vi "test.vi"() -> ()   [LabVIEW 2023]
uses:
  <vilib>/Instr/_visa.llb/VISA Configure Serial Port (Instr).vi
panel:
  out "read buffer 2":string
  out "read buffer":string
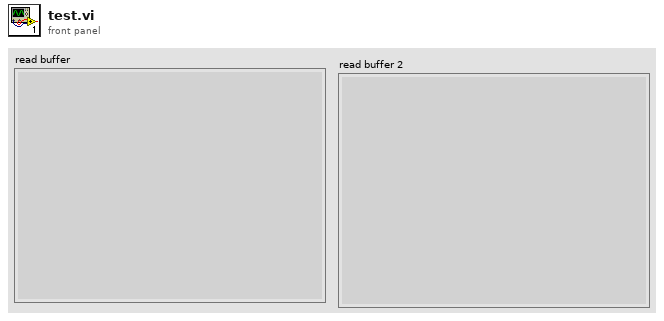
[diagram p1: front panel]
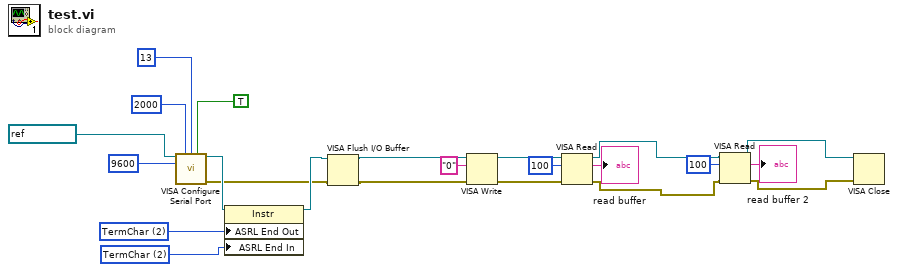
[diagram p0: block diagram]
diagram:
  w18 = u16 2 items=["None", "Last Bit", "TermChar", "Break"] ("Serial Settings:End Mode for Writes")
  w17 = u16 2 items=["None", "Last Bit", "TermChar", "Break"] ("Serial Settings:End Mode for Writes")
  n1 = call-poly "VISA Configure Serial Port"("VISA resource name"=refnum<visa-resource-name> "COM10", "timeout (10sec)"=u32 2000, "termination char\n(0xA = '\\n' = LF)"=u8 13 ("termination char\n(0xA = '\\n' = LF)"), "Enable Termination\nChar (T)"=TRUE ("Enable Termination\nChar (T)"), "baud rate (9600)"=u32 9600) -> ("VISA resource name out"=w19:refnum<visa-resource-name>, "error out"=w2:errorcluster)  [unwired: 9 in]
  n2 = property class="Instr"(reference=w19, "ASRL End Out"=w18, "ASRL End In"=w17) -> (reference out=w5:refnum<visa-resource-name>)  [unwired: 1 in, 1 out]
  n3 = VISA Flush I/O Buffer(VISA resource name=w5, error in (no error)=w2) -> (VISA resource name out=w4:refnum<visa-resource-name>, error out=w3:errorcluster)  [unwired: 1 in]
  n4 = VISA Write(VISA resource name=w4, write buffer="0", error in (no error)=w3) -> (VISA resource name out=w15:refnum<visa-resource-name>, error out=w14:errorcluster)  [unwired: 1 out]
  n5 = VISA Read(VISA resource name=w15, byte count=u32 100, error in (no error)=w14) -> (VISA resource name out=w9:refnum<visa-resource-name>, read buffer=→"read buffer":string, error out=w8:errorcluster)  [unwired: 1 out]
  n6 = VISA Read(VISA resource name=w9, byte count=u32 100, error in (no error)=w8) -> (VISA resource name out=w6:refnum<visa-resource-name>, read buffer=→"read buffer 2":string, error out=w7:errorcluster)  [unwired: 1 out]
  n7 = VISA Close(VISA resource name=w6, error in (no error)=w7) -> ()  [unwired: 1 out]
